vi "460 proj alpha.vi"() -> ()   [LabVIEW 2022 SP3]
uses:
  4060timecase.ctl
  <vilib>/sound2/lvsound2.llb/Sampling Mode.ctl
  4060subcasev2.ctl
  <vilib>/DAQmx/write.llb/DAQmx Write (Digital 1D Bool 1Chan 1Samp).vi
  62f802e7-f2dc-4d8a-a8e5-ab53cfb57c08.vi
  e1d0f7a0-9947-4ad8-8ac9-96135730a529.vi
  715f9e0f-8cb6-4fff-8a35-6535642fb82b.vi
  d1fa0bc4-31c7-44d2-9494-ddc12c5262e6.vi
  e97d7d1c-9cf7-499a-84b2-3041ff66f3d3.vi
  daa3e593-bf9d-4693-a451-b37ae69cdf9d.vi
  ae99be6c-c37c-4ad1-810a-db7e2be311bb.vi
  7a178aea-8366-4402-91cf-f9756686beea.vi
  5c64ab0a-a384-4fd4-873d-7fa8e23df335.vi
  1a855142-eefd-40c8-a2f9-4711cbabd8ad.vi
  aaa2aacd-ac84-4a8d-9874-ed439ef16769.vi
  2e93e64d-414c-47cd-bdfc-17e5d0d425ac.vi
  <vilib>/DAQmx/create/channels.llb/DAQmx Create Channel (DO-Digital Output).vi
  <vilib>/DAQmx/miscellaneous.llb/DAQmx Fill In Error Info.vi
  <vilib>/sound2/lvsound2.llb/Sound File Info (path).vi
  <vilib>/sound2/lvsound2.llb/Sound File Read Open.vi
  <vilib>/sound2/lvsound2.llb/Sound File Read (DBL).vi
  <vilib>/sound2/lvsound2.llb/Sound Output Write (DBL).vi
panel:
  out "error out 51":errorcluster
  out "error out 50":errorcluster
  out "error out 49":errorcluster
  out "error out 48":errorcluster
  out "error out 47":errorcluster
  out "error out 46":errorcluster
  out "error out 45":errorcluster
  out "error out 44":errorcluster
  out "error out 43":errorcluster
  out "error out 42":errorcluster
  out "error out 41":errorcluster
  out "error out 40":errorcluster
  out "error out 39":errorcluster
  in  "Number of Samples/Iteration":i32=2500
  in  "Device ID":u32
  in  "Stop":bool
  out "Current Iteration":i32
  out "Array 3":dbl[](array[numeric])
  out "Waveform Chart":waveform(dbl)[](graph)
  out "Array 7":bool[](array[boolean])
  out "error out 38":errorcluster
  out "error out 29":errorcluster
  out "Boolean 5":bool
  out "error out 25":errorcluster
  out "Boolean 4":bool
  out "Boolean 3":bool
  out "Boolean 2":bool
  out "error out 37":errorcluster
  out "error out 36":errorcluster
  out "error out 35":errorcluster
  out "error out 34":errorcluster
  out "error out 33":errorcluster
  out "error out 32":errorcluster
  out "error out 31":errorcluster
  out "error out 30":errorcluster
  out "error out 28":errorcluster
  out "error out 27":errorcluster
  out "error out 26":errorcluster
  in  "stop 3":bool
  # "I love those J I N G L E Bells\n\nOH\n\nThose Holiday J I N G L E Bells\n\nOH\n\nThose Happy J I N G L E\n\nB E double L S\n\nI love those J I N G L E bells\n\nOH\n\nJingle bells, jingle bells\n\nJingle all the way\n\nOh, what fun it is to ride\n\nIn a one horse open sleigh\n\nJingle bells, jingle bells\n\nJingle all the way\n\nOh, what fun it is to ride\n\nIn a one horse open sleigh\n\nDashing through the snow\n\n(Rudolph)\n\nIn a one horse open sleigh \n\n(Today)\n\nO'er the fields we go\n\n(Rudolph)\n\nLaughing all the way \n\n(Today)\n\nBells on bob-tail ring\n\nBING BING\n\nMakin' our spirits bright\n\nBONG BONG \n\nWhat fun it is to ride and sing\n\nA sleighin' song tonight\n\nHO HO HO\n\nHO HO HO\n\nHO HO HO HO HO\n\nHO HO HO HO HO HO HO\n \nHO HO HO HO HO HO\n\nJingle bells, jingle bells\n\nJingle all the way\n\nOh, what fun it is to ride\n\nIn a one horse open sleigh\n\nI love those J I N G L E Bells\n\nOH\n\nThose Holiday J I N G L E Bells\n\nOH\n\nThose Happy J I N G L E\n\nB E double L S\n\nI love those jingle bells\n\nAll the way!\n\nJingle all the\n\nWayyyyyyyyyy!"
  # "1. (v1)  0, 2, 4, (0 2 4 6), (1 3 5 7), (0 2 4 6), (1 3 5 7), (0 2 4 6), (1 3 5 7), off, \n\n(v1) LIGHTS\n\n(v2) 7, 5, 3, 1,  (1 3 5 7),  (0 2 4 6), (1 3 5 7),  (0 2 4 6),(1 3 5 7),  (0 2 4 6), off\n\n(v2) LIGHTS\n\n(v3)  0, 2, 4, (0 2 4 6), (1 3 5 7), (0 2 4 6), (1 3 5 7), (0 2 4 6), (1 3 5 7), off,\n\n2. (v4) (0 1), (7 6), off, (2 3), (4 5)\n\n(v5)  0, 2, 4, (0 2 4 6), (1 3 5 7), (0 2 4 6), (1 3 5 7), (0 2 4 6), (1 3 5 7), off\n\n(v6) LIGHTS"
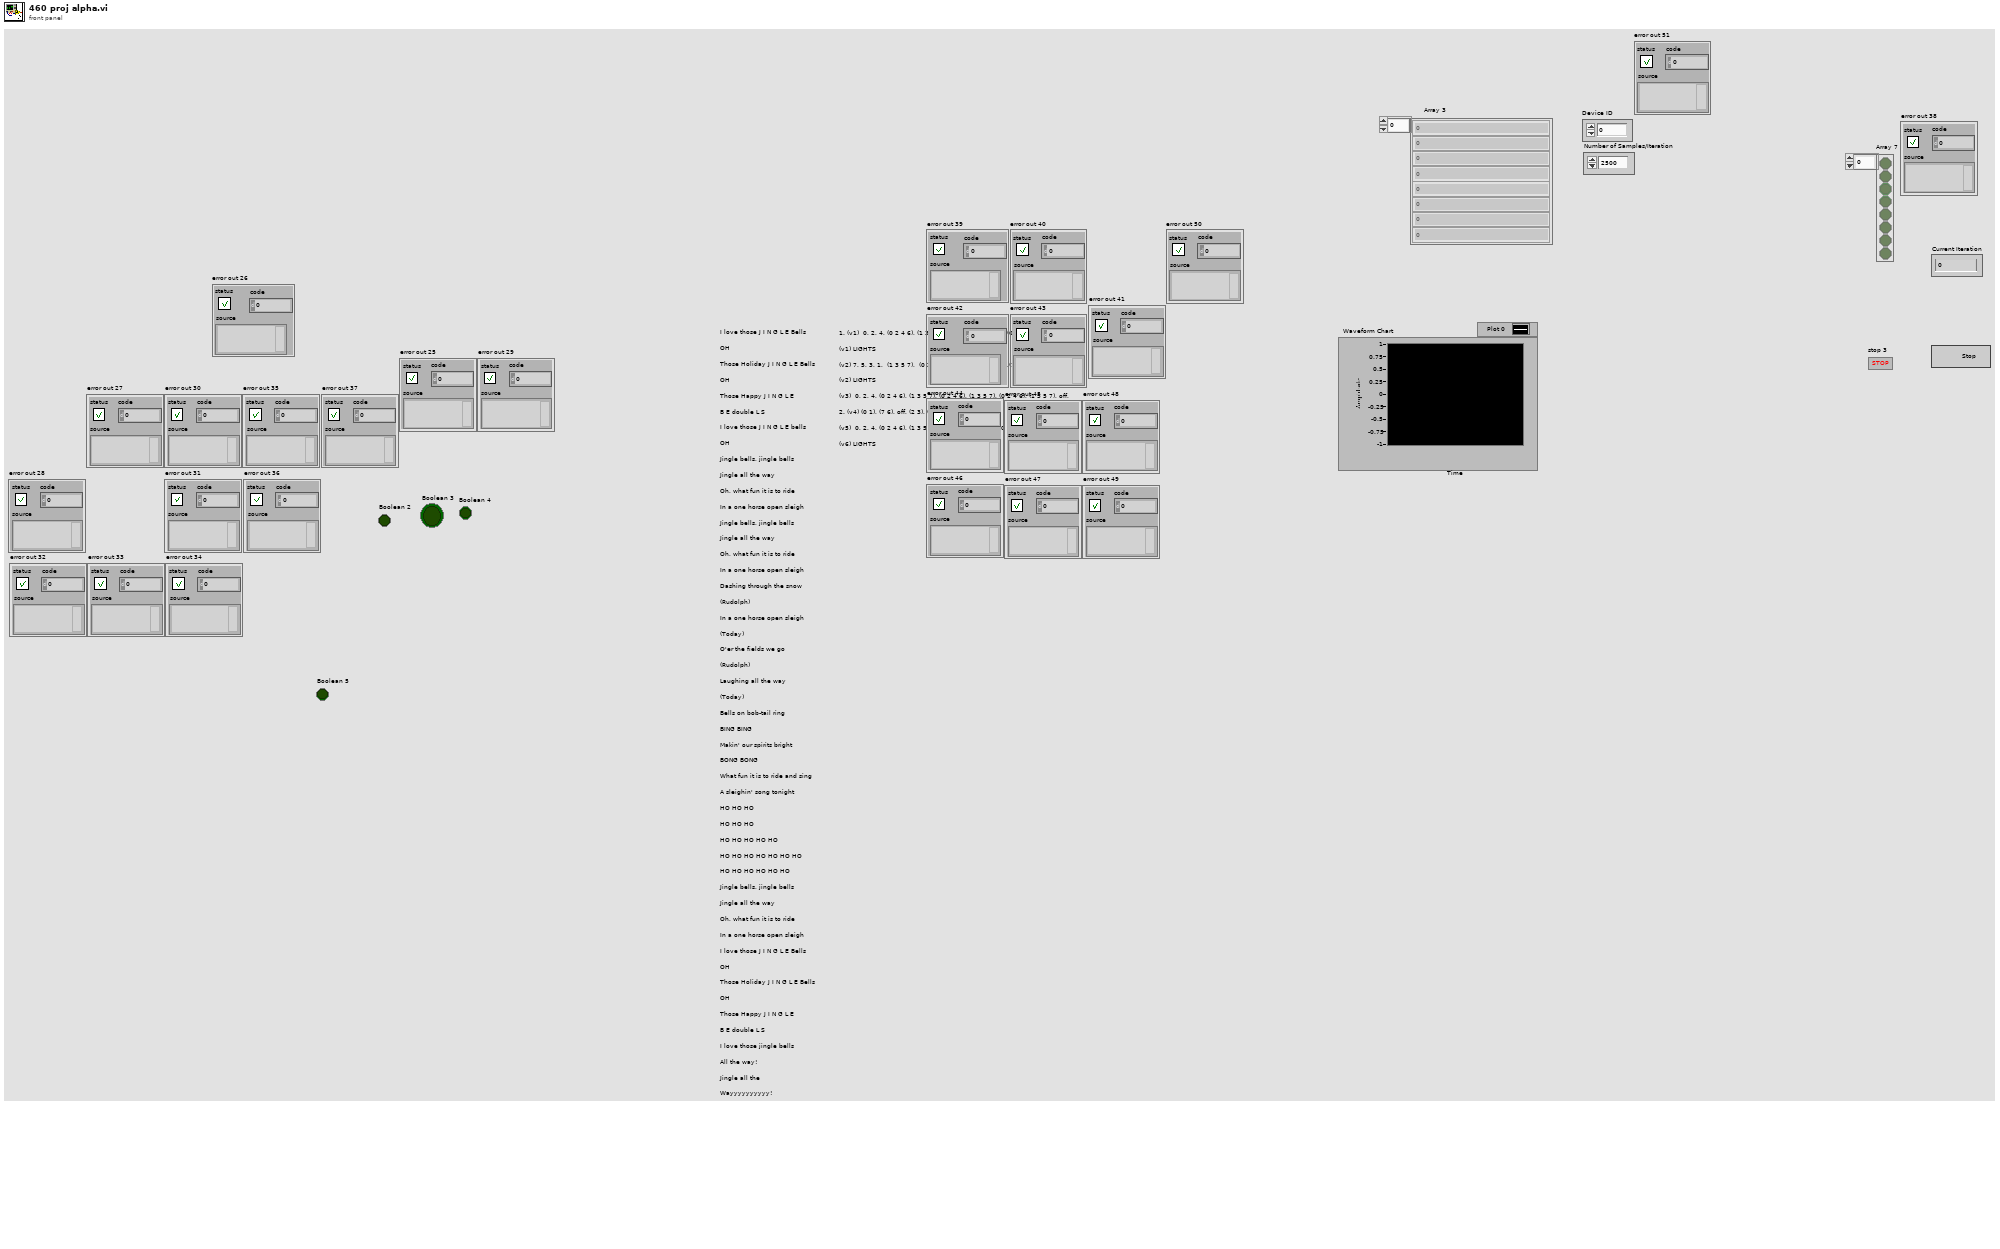
[diagram p1: front panel]
types:
  T1 = typedef "Sampling Mode.ctl" = i32
  T2 = typedef "4060timecase.ctl" = enum16{"v1-I love those", "v1-J", "v1-I", "v1-N", "v1-G", "v1-L", "v1-E", "v1-Bells", "v1-OH", "v1-OHoff", "v2-those holiday", "v2-J", "v2-I", "v2-N", "v2-G", "v2-L", "v2-E", "v2-Bells", "v2-OH", "v2-OHoff", "v3-those happy", "v3-J", "v3-I", "v3-N", "v3-G", "v3-L", "v3-E", "v4-B", "v4-E", "v4-double", "v4-L", "v4-S", "v4-Soff", "v5-I love those", "v5-J", "v5-I", "v5-N", "v5-G", "v5-L", "v5-E", "v5-Bells", "v5-OH", "v1-end"}
  T3 = typedef "4060subcasev2.ctl" = enum16{"v4 B", "v4 E", "v4 double", "v4 L", "v4 S", "v3 those happy", "off", "(0 2 4 6)", "LIGHTS", "(1 3 5 7)", "v1 I love those", "v2 those holiday"}
  T4 = typedef "Sound Data Format.ctl" = cluster{"sample rate (S/s)":dbl, "number of channels":i32, "bits per sample":i32}
  T5 = typedef "Sound File Refnum.ctl" = refnum<file>
  T6 = typedef "Sound Output Task ID.ctl" = u32
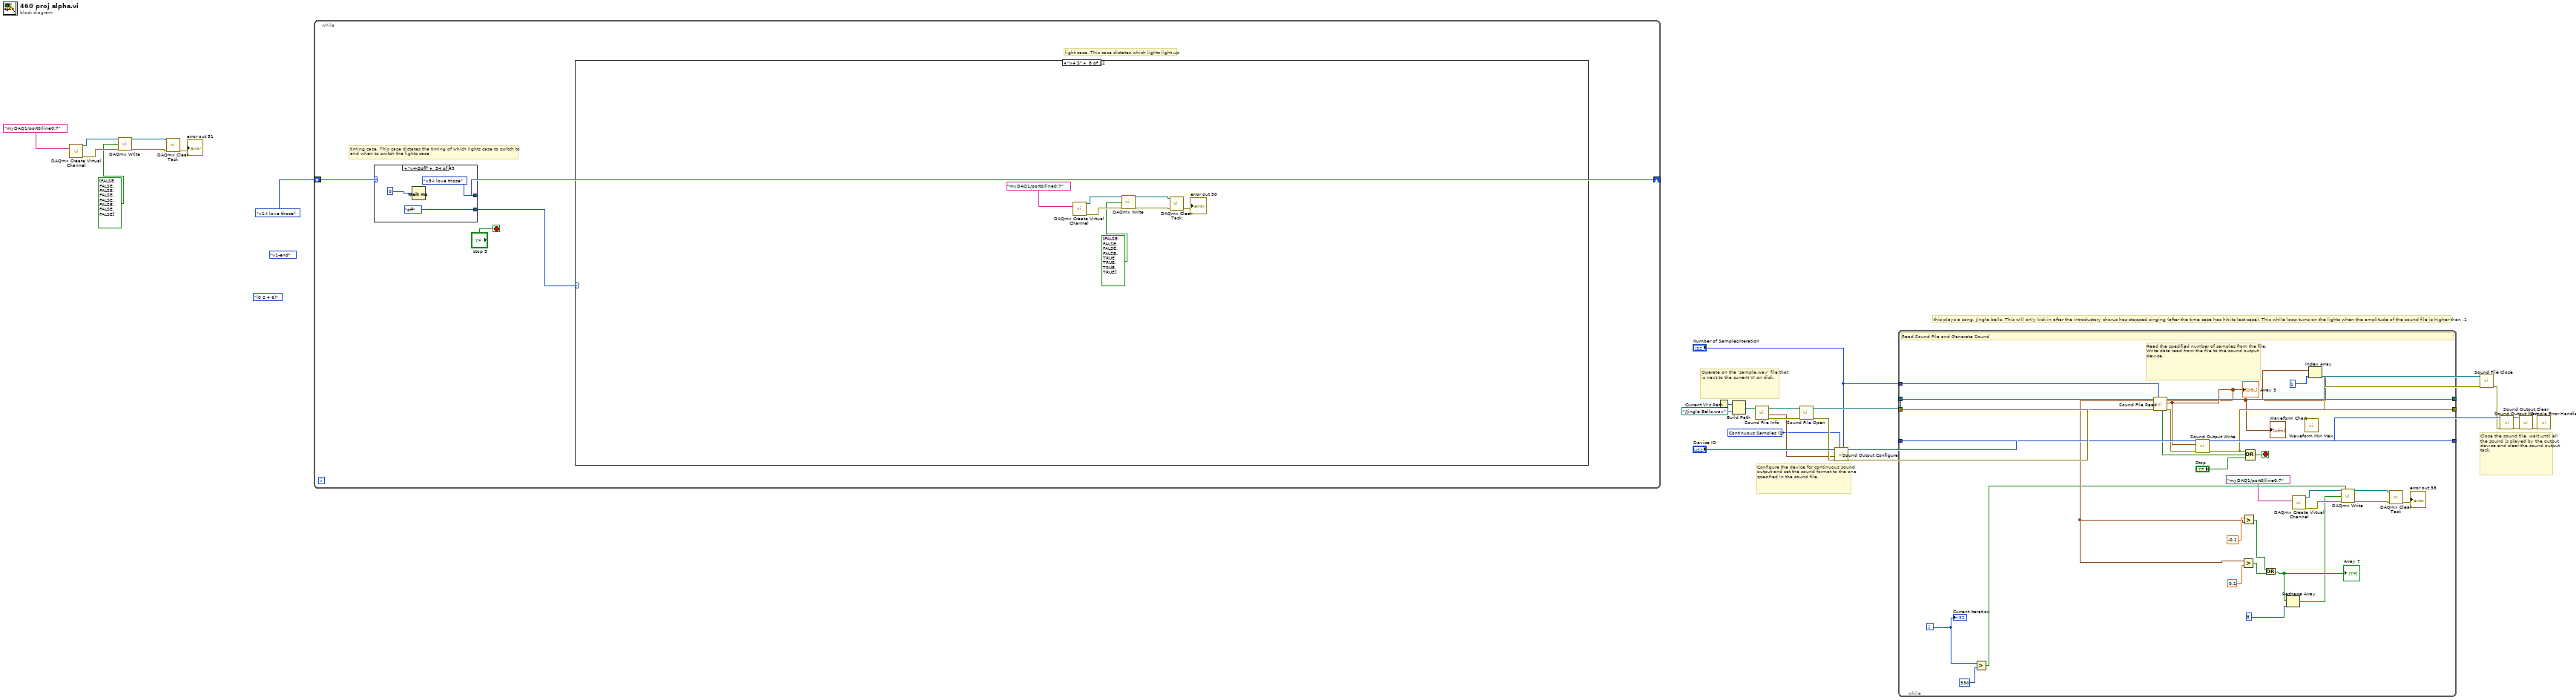
[diagram p0: block diagram]
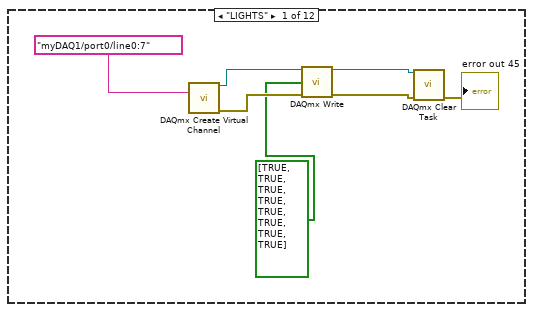
[diagram p2: hidden frame]
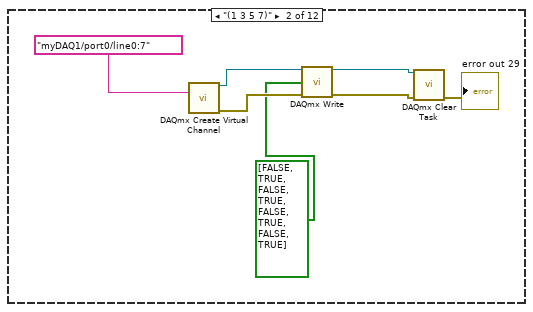
[diagram p3: hidden frame]
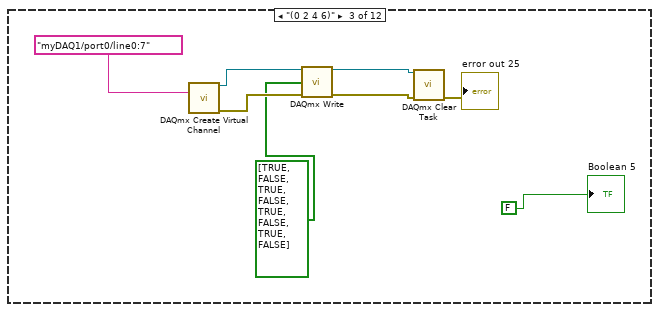
[diagram p4: hidden frame]
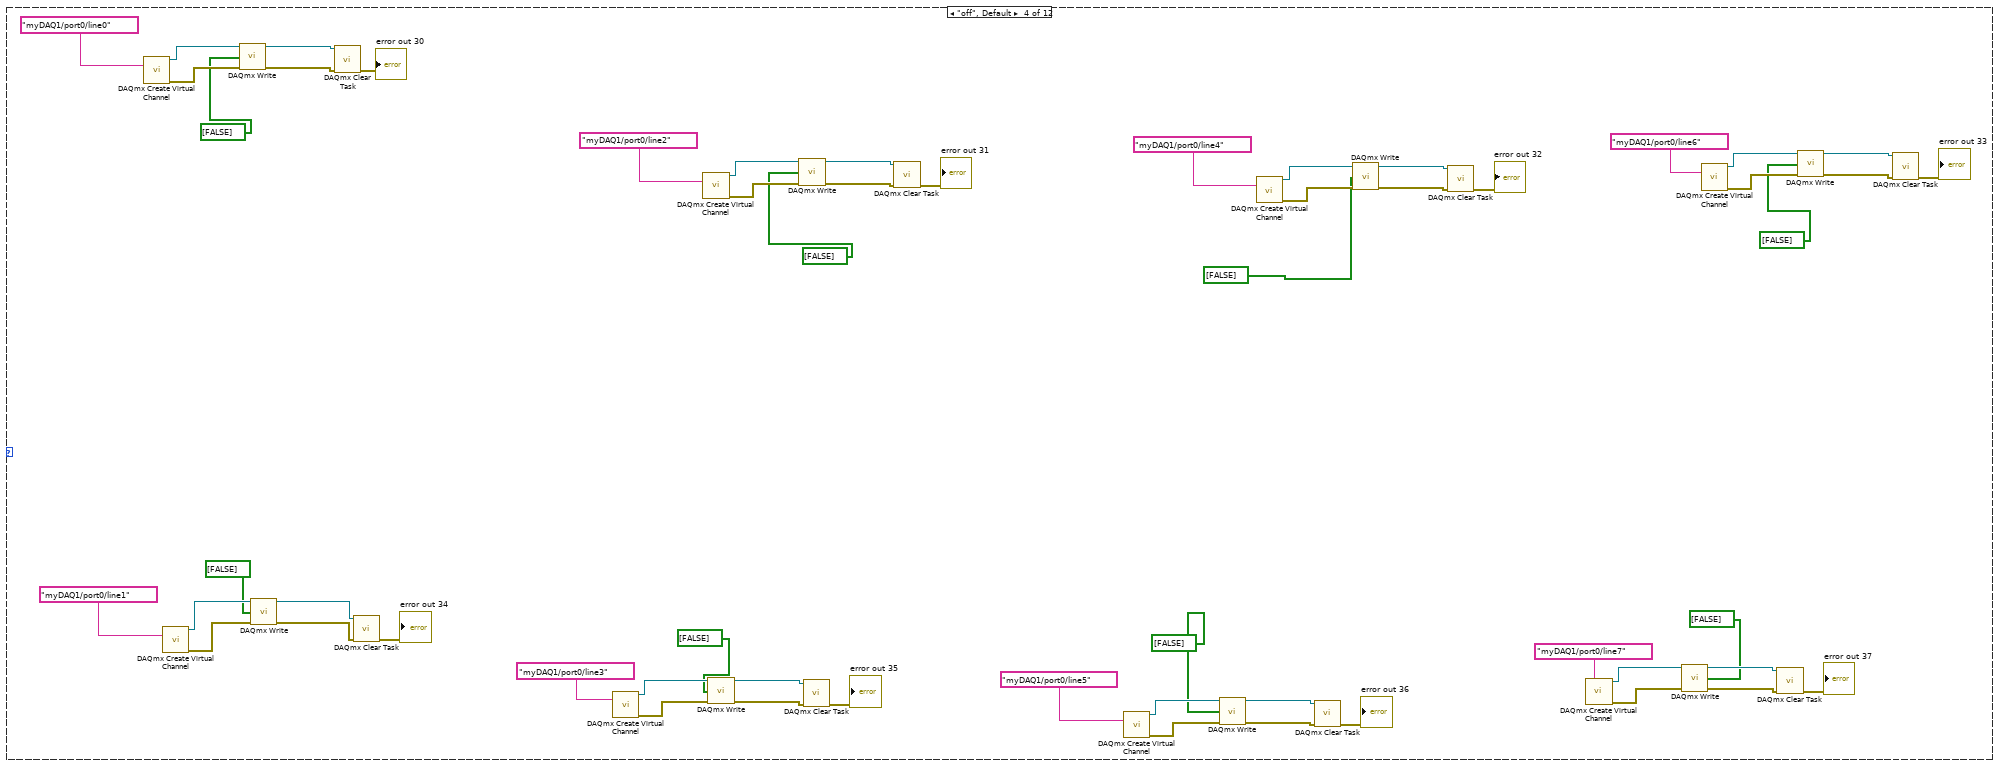
[diagram p5: hidden frame]
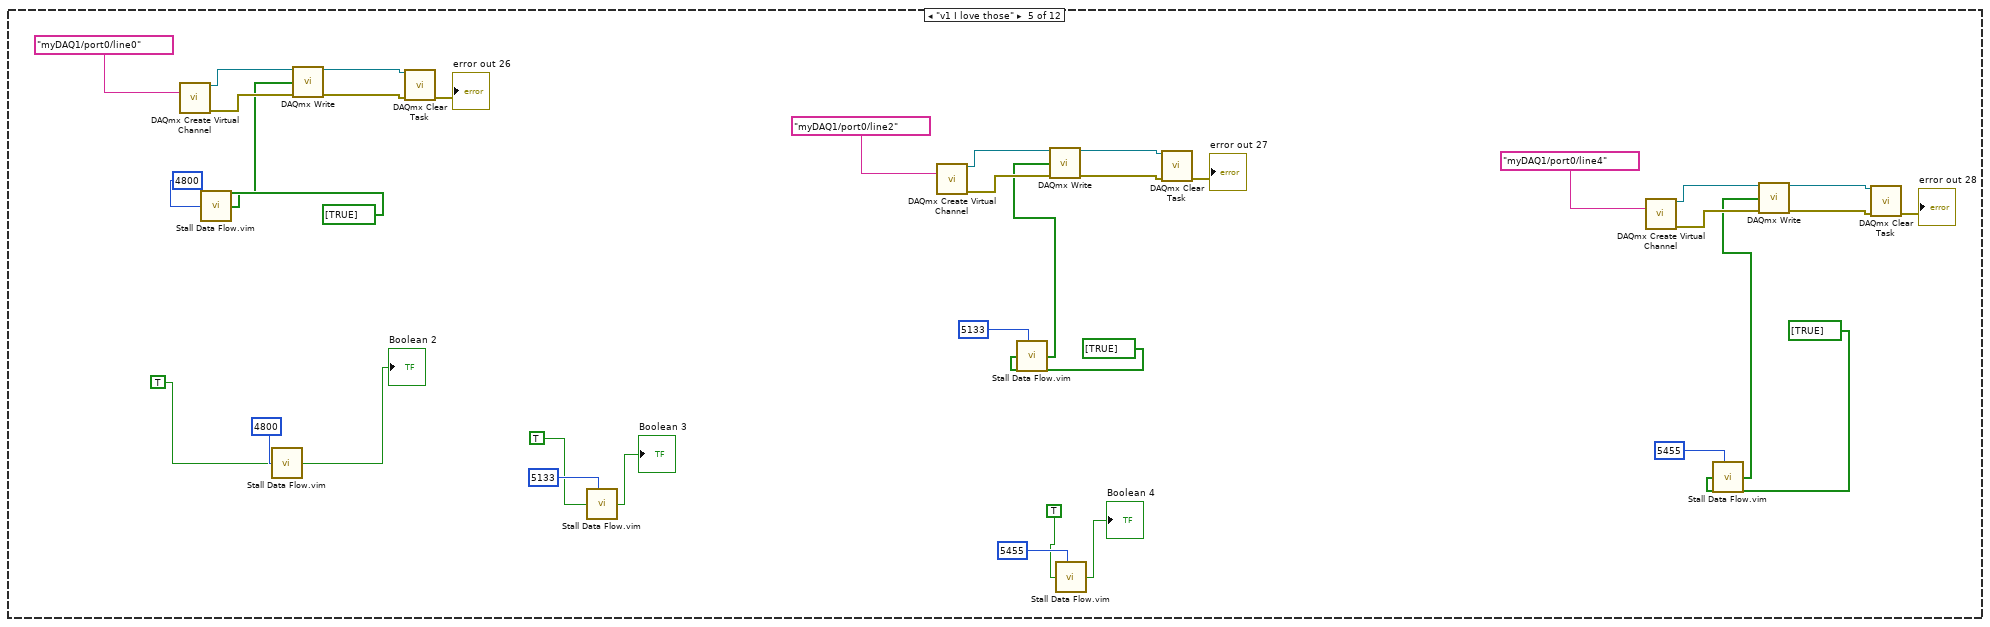
[diagram p6: hidden frame]
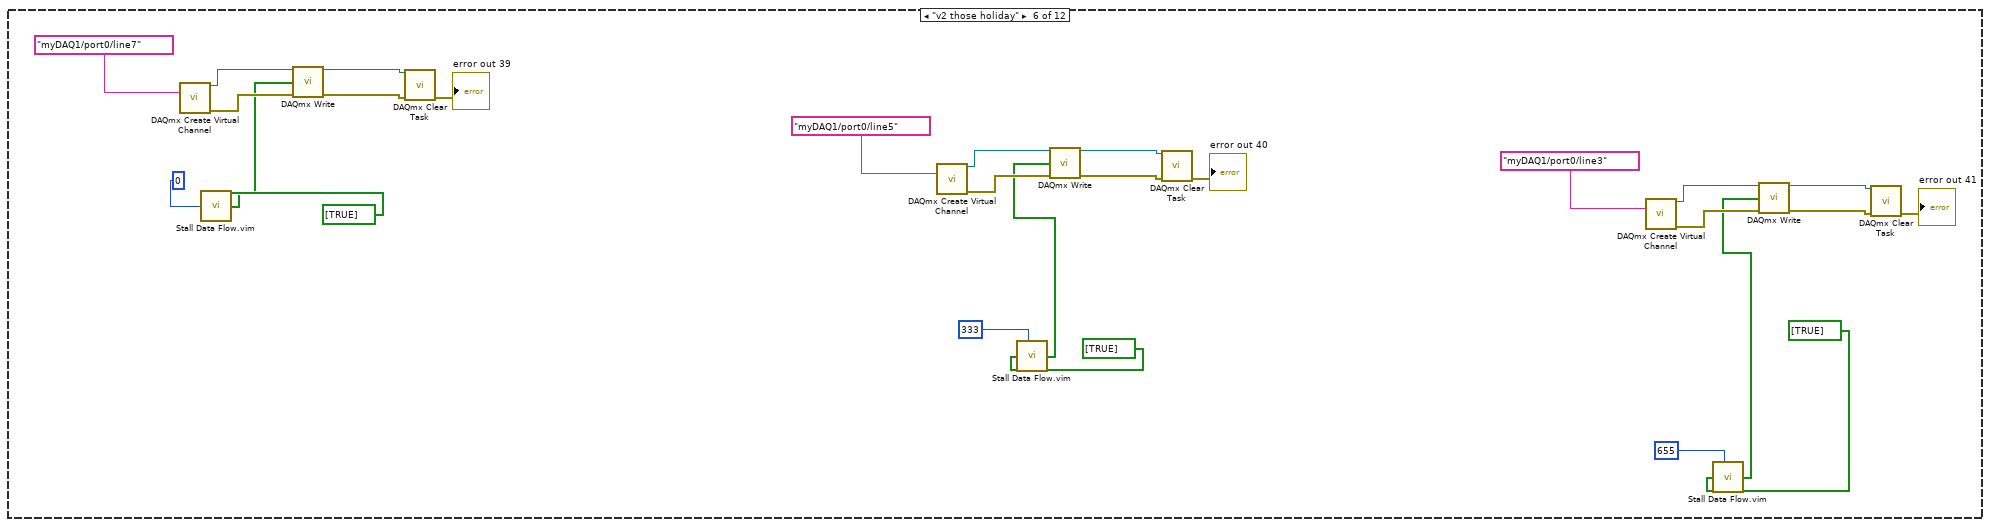
[diagram p7: hidden frame]
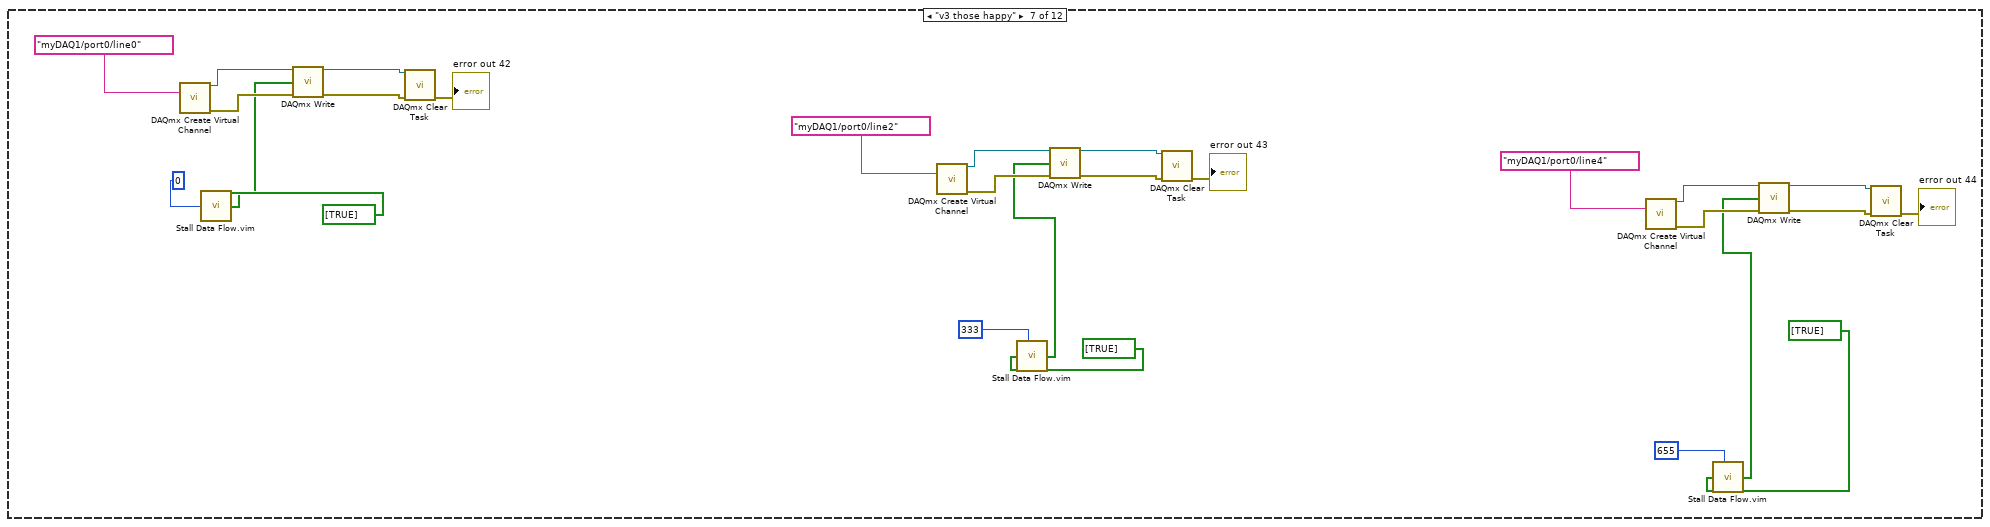
[diagram p8: hidden frame]
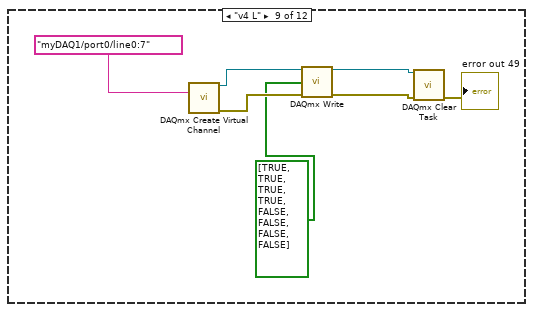
[diagram p9: hidden frame]
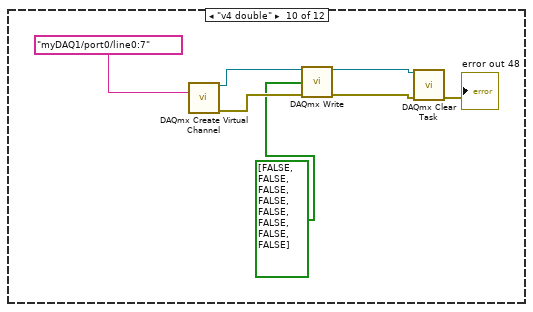
[diagram p10: hidden frame]
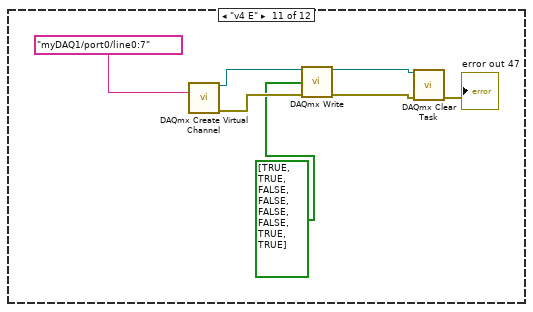
[diagram p11: hidden frame]
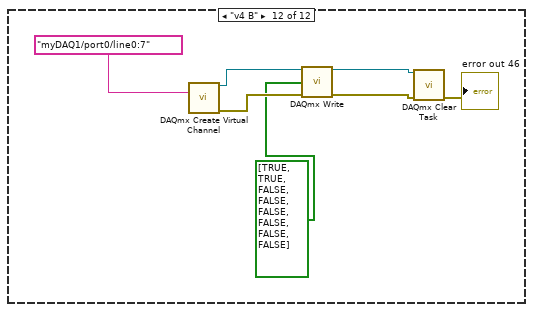
[diagram p12: hidden frame]
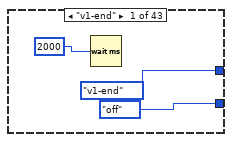
[diagram p13: hidden frame]
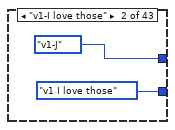
[diagram p14: hidden frame]
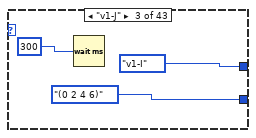
[diagram p15: hidden frame]
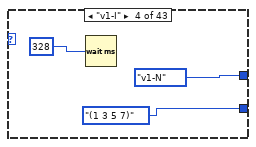
[diagram p16: hidden frame]
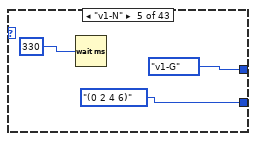
[diagram p17: hidden frame]
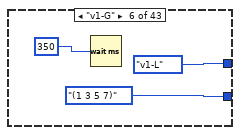
[diagram p18: hidden frame]
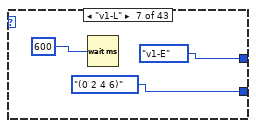
[diagram p19: hidden frame]
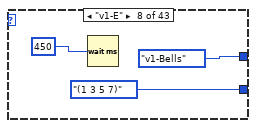
[diagram p20: hidden frame]
diagram:
  w12 = T1 1 items=["Finite Samples", "Continuous Samples"] ("sample mode")
  (unwired) 4060timecase."v1-end"
  (unwired) 4060subcasev2."(0 2 4 6)"
  # "this plays a song, Jingle bells. This will only kick in after the introductory chorus has stopped singing (after the time case has hit its last case). This while loop turns on the lights when the amplitude of the sound file is higher than .1"
  # "Operate on the 'sample.wav' file that is next to the current VI on disk."
  # "Close the sound file, wait until all the sound is played by the output device and clear the sound output task."
  # "Configure the device for continuous sound output and set the sound format to the one specified in the sound file."
  n1 = call-poly <vilib>:"DAQmx Create Virtual Channel.vi"("lines"=tag "myDAQ1/port0/line0:7") -> ("task out"=w7:refnum<k21>, "error out"=w5:errorcluster)  [unwired: 13 in]
  n2 = call-poly <vilib>:"DAQmx Write.vi"("task/channels in"=w7, "data"=bool[] [FALSE, FALSE, FALSE, FALSE, FALSE, FALSE, FALSE, FALSE], "error in"=w5) -> ("task out"=w6:refnum<k21>, "error out"=w4:errorcluster)  [unwired: 10 in, 1 out]
  n3 = call <vilib>:"DAQmx Clear Task.vi"("task in"=w6, "error in"=w4) -> ("error out"=→"error out 51":errorcluster)  [unwired: 13 in]
  n4 = while {
    shift-right: [w30] -> _
    shift-left: 4060timecase."v1-I love those" -> [w32]
    stop <- "stop 3" stop-if-true
    # "light case. This case dictates which lights light up"
    # "timing case. This case dictates the timing of which lights case to switch to\nand when to switch the lights case"
    n5 = case shown="\"v4-Soff\"" w32 {
      tunnel: [4060subcasev2."off" 4060subcasev2."v1 I love those" 4060subcasev2."(0 2 4 6)" 4060subcasev2."(1 3 5 7)" 4060subcasev2."(0 2 4 6)" 4060subcasev2."(1 3 5 7)" 4060subcasev2."(0 2 4 6)" 4060subcasev2."(1 3 5 7)" 4060subcasev2."off" 4060subcasev2."LIGHTS" 4060subcasev2."off" 4060subcasev2."v2 those holiday" 4060subcasev2."(1 3 5 7)" 4060subcasev2."(0 2 4 6)" 4060subcasev2."(1 3 5 7)" 4060subcasev2."(0 2 4 6)" 4060subcasev2."(1 3 5 7)" 4060subcasev2."(0 2 4 6)" 4060subcasev2."off" 4060subcasev2."LIGHTS" 4060subcasev2."off" 4060subcasev2."v3 those happy" 4060subcasev2."(0 2 4 6)" 4060subcasev2."(1 3 5 7)" 4060subcasev2."(0 2 4 6)" 4060subcasev2."(1 3 5 7)" 4060subcasev2."(0 2 4 6)" 4060subcasev2."(1 3 5 7)" 4060subcasev2."v4 B" 4060subcasev2."v4 E" 4060subcasev2."v4 double" 4060subcasev2."v4 L" 4060subcasev2."v4 S" 4060subcasev2."off" 4060subcasev2."v2 those holiday" 4060subcasev2."(1 3 5 7)" 4060subcasev2."(0 2 4 6)" 4060subcasev2."(1 3 5 7)" 4060subcasev2."(0 2 4 6)" 4060subcasev2."(1 3 5 7)" 4060subcasev2."(0 2 4 6)" 4060subcasev2."off" 4060subcasev2."LIGHTS"] -> w29
      tunnel: [4060timecase."v1-end" 4060timecase."v1-J" 4060timecase."v1-I" 4060timecase."v1-N" 4060timecase."v1-G" 4060timecase."v1-L" 4060timecase."v1-E" 4060timecase."v1-Bells" 4060timecase."v1-OH" 4060timecase."v1-OHoff" 4060timecase."v2-those holiday" 4060timecase."v2-J" 4060timecase."v2-I" 4060timecase."v2-N" 4060timecase."v2-G" 4060timecase."v2-L" 4060timecase."v2-E" 4060timecase."v2-Bells" 4060timecase."v2-OH" 4060timecase."v2-OHoff" 4060timecase."v3-those happy" 4060timecase."v3-J" 4060timecase."v3-I" 4060timecase."v3-N" 4060timecase."v3-G" 4060timecase."v3-L" 4060timecase."v3-E" 4060timecase."v4-B" 4060timecase."v4-E" 4060timecase."v4-double" 4060timecase."v4-L" 4060timecase."v4-S" 4060timecase."v4-Soff" 4060timecase."v5-I love those" 4060timecase."v5-J" 4060timecase."v5-I" 4060timecase."v5-N" 4060timecase."v5-G" 4060timecase."v5-L" 4060timecase."v5-E" 4060timecase."v5-Bells" 4060timecase."v5-OH" 4060timecase."v1-end"] -> w30
      frame "v1-end" {
        n6 = Wait (ms)(milliseconds to wait=2000) -> ()  [unwired: 1 out]
      }
      frame "v1-I love those" {
      }
      frame "v1-J" {
        n7 = Wait (ms)(milliseconds to wait=300) -> ()  [unwired: 1 out]
      }
      frame "v1-I" {
        n8 = Wait (ms)(milliseconds to wait=328) -> ()  [unwired: 1 out]
      }
      frame "v1-N" {
        n9 = Wait (ms)(milliseconds to wait=330) -> ()  [unwired: 1 out]
      }
      frame "v1-G" {
        n10 = Wait (ms)(milliseconds to wait=350) -> ()  [unwired: 1 out]
      }
      frame "v1-L" {
        n11 = Wait (ms)(milliseconds to wait=600) -> ()  [unwired: 1 out]
      }
      frame "v1-E" {
        n12 = Wait (ms)(milliseconds to wait=450) -> ()  [unwired: 1 out]
      }
      frame "v1-Bells" {
        n13 = Wait (ms)(milliseconds to wait=330) -> ()  [unwired: 1 out]
      }
      frame "v1-OH" {
        n14 = Wait (ms)(milliseconds to wait=1000) -> ()  [unwired: 1 out]
      }
      frame "v1-OHoff" {
        n15 = Wait (ms)(milliseconds to wait=300) -> ()  [unwired: 1 out]
      }
      frame "v2-those holiday" {
        n16 = Wait (ms)(milliseconds to wait=500) -> ()  [unwired: 1 out]
      }
      frame "v2-J" {
        n17 = Wait (ms)(milliseconds to wait=300) -> ()  [unwired: 1 out]
      }
      frame "v2-I" {
        n18 = Wait (ms)(milliseconds to wait=328) -> ()  [unwired: 1 out]
      }
      frame "v2-N" {
        n19 = Wait (ms)(milliseconds to wait=330) -> ()  [unwired: 1 out]
      }
      frame "v2-G" {
        n20 = Wait (ms)(milliseconds to wait=350) -> ()  [unwired: 1 out]
      }
      frame "v2-L" {
        n21 = Wait (ms)(milliseconds to wait=600) -> ()  [unwired: 1 out]
      }
      frame "v2-E" {
        n22 = Wait (ms)(milliseconds to wait=450) -> ()  [unwired: 1 out]
      }
      frame "v2-Bells" {
        n23 = Wait (ms)(milliseconds to wait=330) -> ()  [unwired: 1 out]
      }
      frame "v2-OH" {
        n24 = Wait (ms)(milliseconds to wait=1000) -> ()  [unwired: 1 out]
      }
      frame "v2-OHoff" {
        n25 = Wait (ms)(milliseconds to wait=300) -> ()  [unwired: 1 out]
      }
      frame "v3-those happy" {
        n26 = Wait (ms)(milliseconds to wait=330) -> ()  [unwired: 1 out]
      }
      frame "v3-J" {
        n27 = Wait (ms)(milliseconds to wait=330) -> ()  [unwired: 1 out]
      }
      frame "v3-I" {
        n28 = Wait (ms)(milliseconds to wait=328) -> ()  [unwired: 1 out]
      }
      frame "v3-N" {
        n29 = Wait (ms)(milliseconds to wait=330) -> ()  [unwired: 1 out]
      }
      frame "v3-G" {
        n30 = Wait (ms)(milliseconds to wait=350) -> ()  [unwired: 1 out]
      }
      frame "v3-L" {
        n31 = Wait (ms)(milliseconds to wait=600) -> ()  [unwired: 1 out]
      }
      frame "v3-E" {
        n32 = Wait (ms)(milliseconds to wait=450) -> ()  [unwired: 1 out]
      }
      frame "v4-B" {
        n33 = Wait (ms)(milliseconds to wait=1000) -> ()  [unwired: 1 out]
      }
      frame "v4-E" {
        n34 = Wait (ms)(milliseconds to wait=330) -> ()  [unwired: 1 out]
      }
      frame "v4-double" {
        n35 = Wait (ms)(milliseconds to wait=330) -> ()  [unwired: 1 out]
      }
      frame "v4-L" {
        n36 = Wait (ms)(milliseconds to wait=330) -> ()  [unwired: 1 out]
      }
      frame "v4-S" {
        n37 = Wait (ms)(milliseconds to wait=330) -> ()  [unwired: 1 out]
      }
      frame "v4-Soff" {
        n38 = Wait (ms)(milliseconds to wait=0) -> ()  [unwired: 1 out]
      }
      frame "v5-I love those" {
        n39 = Wait (ms)(milliseconds to wait=330) -> ()  [unwired: 1 out]
      }
      frame "v5-J" {
        n40 = Wait (ms)(milliseconds to wait=330) -> ()  [unwired: 1 out]
      }
      frame "v5-I" {
        n41 = Wait (ms)(milliseconds to wait=330) -> ()  [unwired: 1 out]
      }
      frame "v5-N" {
        n42 = Wait (ms)(milliseconds to wait=330) -> ()  [unwired: 1 out]
      }
      frame "v5-G" {
        n43 = Wait (ms)(milliseconds to wait=330) -> ()  [unwired: 1 out]
      }
      frame "v5-L" {
        n44 = Wait (ms)(milliseconds to wait=330) -> ()  [unwired: 1 out]
      }
      frame "v5-E" {
        n45 = Wait (ms)(milliseconds to wait=330) -> ()  [unwired: 1 out]
      }
      frame "v5-Bells" {
        n46 = Wait (ms)(milliseconds to wait=330) -> ()  [unwired: 1 out]
      }
      frame "v5-OH" {
        n47 = Wait (ms)(milliseconds to wait=330) -> ()  [unwired: 1 out]
      }
    }
    n48 = case shown="\"v4 S\"" w29 {
      frame "LIGHTS" {
        n49 = call-poly <vilib>:"DAQmx Create Virtual Channel.vi"("lines"=tag "myDAQ1/port0/line0:7") -> ("task out"=w39:refnum<k21>, "error out"=w37:errorcluster)  [unwired: 13 in]
        n50 = call-poly <vilib>:"DAQmx Write.vi"("task/channels in"=w39, "data"=bool[] [TRUE, TRUE, TRUE, TRUE, TRUE, TRUE, TRUE, TRUE], "error in"=w37) -> ("task out"=w38:refnum<k21>, "error out"=w36:errorcluster)  [unwired: 10 in, 1 out]
        n51 = call <vilib>:"DAQmx Clear Task.vi"("task in"=w38, "error in"=w36) -> ("error out"=→"error out 45":errorcluster)  [unwired: 13 in]
      }
      frame "(1 3 5 7)" {
        n52 = call-poly <vilib>:"DAQmx Create Virtual Channel.vi"("lines"=tag "myDAQ1/port0/line0:7") -> ("task out"=w46:refnum<k21>, "error out"=w44:errorcluster)  [unwired: 13 in]
        n53 = call-poly <vilib>:"DAQmx Write.vi"("task/channels in"=w46, "data"=bool[] [FALSE, TRUE, FALSE, TRUE, FALSE, TRUE, FALSE, TRUE], "error in"=w44) -> ("task out"=w45:refnum<k21>, "error out"=w43:errorcluster)  [unwired: 10 in, 1 out]
        n54 = call <vilib>:"DAQmx Clear Task.vi"("task in"=w45, "error in"=w43) -> ("error out"=→"error out 29":errorcluster)  [unwired: 13 in]
      }
      frame "(0 2 4 6)" {
        n55 = call-poly <vilib>:"DAQmx Create Virtual Channel.vi"("lines"=tag "myDAQ1/port0/line0:7") -> ("task out"=w54:refnum<k21>, "error out"=w52:errorcluster)  [unwired: 13 in]
        n56 = call-poly <vilib>:"DAQmx Write.vi"("task/channels in"=w54, "data"=bool[] [TRUE, FALSE, TRUE, FALSE, TRUE, FALSE, TRUE, FALSE], "error in"=w52) -> ("task out"=w53:refnum<k21>, "error out"=w51:errorcluster)  [unwired: 10 in, 1 out]
        n57 = call <vilib>:"DAQmx Clear Task.vi"("task in"=w53, "error in"=w51) -> ("error out"=→"error out 25":errorcluster)  [unwired: 13 in]
        "Boolean 5" <- FALSE
      }
      frame "off", Default {
        n58 = call-poly <vilib>:"DAQmx Create Virtual Channel.vi"("lines"=tag "myDAQ1/port0/line0") -> ("task out"=w110:refnum<k21>, "error out"=w108:errorcluster)  [unwired: 13 in]
        n59 = call-poly <vilib>:"DAQmx Create Virtual Channel.vi"("lines"=tag "myDAQ1/port0/line1") -> ("task out"=w86:refnum<k21>, "error out"=w84:errorcluster)  [unwired: 13 in]
        n60 = call-poly <vilib>:"DAQmx Write.vi"("task/channels in"=w110, "data"=bool[] [FALSE], "error in"=w108) -> ("task out"=w109:refnum<k21>, "error out"=w107:errorcluster)  [unwired: 10 in, 1 out]
        n61 = call-poly <vilib>:"DAQmx Write.vi"("task/channels in"=w86, "data"=bool[] [FALSE], "error in"=w84) -> ("task out"=w85:refnum<k21>, "error out"=w83:errorcluster)  [unwired: 10 in, 1 out]
        n62 = call <vilib>:"DAQmx Clear Task.vi"("task in"=w109, "error in"=w107) -> ("error out"=→"error out 30":errorcluster)  [unwired: 13 in]
        n63 = call <vilib>:"DAQmx Clear Task.vi"("task in"=w85, "error in"=w83) -> ("error out"=→"error out 34":errorcluster)  [unwired: 13 in]
        n64 = call-poly <vilib>:"DAQmx Create Virtual Channel.vi"("lines"=tag "myDAQ1/port0/line3") -> ("task out"=w80:refnum<k21>, "error out"=w78:errorcluster)  [unwired: 13 in]
        n65 = call-poly <vilib>:"DAQmx Create Virtual Channel.vi"("lines"=tag "myDAQ1/port0/line2") -> ("task out"=w104:refnum<k21>, "error out"=w102:errorcluster)  [unwired: 13 in]
        n66 = call-poly <vilib>:"DAQmx Write.vi"("task/channels in"=w80, "data"=bool[] [FALSE], "error in"=w78) -> ("task out"=w79:refnum<k21>, "error out"=w77:errorcluster)  [unwired: 10 in, 1 out]
        n67 = call-poly <vilib>:"DAQmx Write.vi"("task/channels in"=w104, "data"=bool[] [FALSE], "error in"=w102) -> ("task out"=w103:refnum<k21>, "error out"=w101:errorcluster)  [unwired: 10 in, 1 out]
        n68 = call <vilib>:"DAQmx Clear Task.vi"("task in"=w79, "error in"=w77) -> ("error out"=→"error out 35":errorcluster)  [unwired: 13 in]
        n69 = call <vilib>:"DAQmx Clear Task.vi"("task in"=w103, "error in"=w101) -> ("error out"=→"error out 31":errorcluster)  [unwired: 13 in]
        n70 = call-poly <vilib>:"DAQmx Create Virtual Channel.vi"("lines"=tag "myDAQ1/port0/line5") -> ("task out"=w74:refnum<k21>, "error out"=w72:errorcluster)  [unwired: 13 in]
        n71 = call-poly <vilib>:"DAQmx Write.vi"("task/channels in"=w74, "data"=bool[] [FALSE], "error in"=w72) -> ("task out"=w73:refnum<k21>, "error out"=w71:errorcluster)  [unwired: 10 in, 1 out]
        n72 = call-poly <vilib>:"DAQmx Create Virtual Channel.vi"("lines"=tag "myDAQ1/port0/line4") -> ("task out"=w98:refnum<k21>, "error out"=w96:errorcluster)  [unwired: 13 in]
        n73 = call <vilib>:"DAQmx Clear Task.vi"("task in"=w73, "error in"=w71) -> ("error out"=→"error out 36":errorcluster)  [unwired: 13 in]
        n74 = call-poly <vilib>:"DAQmx Write.vi"("task/channels in"=w98, "data"=bool[] [FALSE], "error in"=w96) -> ("task out"=w97:refnum<k21>, "error out"=w95:errorcluster)  [unwired: 10 in, 1 out]
        n75 = call <vilib>:"DAQmx Clear Task.vi"("task in"=w97, "error in"=w95) -> ("error out"=→"error out 32":errorcluster)  [unwired: 13 in]
        n76 = call-poly <vilib>:"DAQmx Create Virtual Channel.vi"("lines"=tag "myDAQ1/port0/line7") -> ("task out"=w68:refnum<k21>, "error out"=w66:errorcluster)  [unwired: 13 in]
        n77 = call-poly <vilib>:"DAQmx Write.vi"("task/channels in"=w68, "data"=bool[] [FALSE], "error in"=w66) -> ("task out"=w67:refnum<k21>, "error out"=w65:errorcluster)  [unwired: 10 in, 1 out]
        n78 = call-poly <vilib>:"DAQmx Create Virtual Channel.vi"("lines"=tag "myDAQ1/port0/line6") -> ("task out"=w92:refnum<k21>, "error out"=w90:errorcluster)  [unwired: 13 in]
        n79 = call <vilib>:"DAQmx Clear Task.vi"("task in"=w67, "error in"=w65) -> ("error out"=→"error out 37":errorcluster)  [unwired: 13 in]
        n80 = call-poly <vilib>:"DAQmx Write.vi"("task/channels in"=w92, "data"=bool[] [FALSE], "error in"=w90) -> ("task out"=w91:refnum<k21>, "error out"=w89:errorcluster)  [unwired: 10 in, 1 out]
        n81 = call <vilib>:"DAQmx Clear Task.vi"("task in"=w91, "error in"=w89) -> ("error out"=→"error out 33":errorcluster)  [unwired: 13 in]
      }
      frame "v1 I love those" {
        n82 = call-poly <vilib>:"DAQmx Create Virtual Channel.vi"("lines"=tag "myDAQ1/port0/line0") -> ("task out"=w146:refnum<k21>, "error out"=w144:errorcluster)  [unwired: 13 in]
        n83 = call "Stall Data Flow.vim"("value in"=bool[] [TRUE], "milliseconds to wait"=4800) -> ("value out"=w117:bool[])  [unwired: 1 out]
        n84 = call "Stall Data Flow.vim"("value in"=TRUE, "milliseconds to wait"=4800) -> ("value out"=→"Boolean 2":bool)  [unwired: 1 out]
        n85 = call-poly <vilib>:"DAQmx Write.vi"("task/channels in"=w146, "data"=w117, "error in"=w144) -> ("task out"=w145:refnum<k21>, "error out"=w143:errorcluster)  [unwired: 10 in, 1 out]
        n86 = call <vilib>:"DAQmx Clear Task.vi"("task in"=w145, "error in"=w143) -> ("error out"=→"error out 26":errorcluster)  [unwired: 13 in]
        n87 = call "Stall Data Flow.vim"("value in"=TRUE, "milliseconds to wait"=5133) -> ("value out"=→"Boolean 3":bool)  [unwired: 1 out]
        n88 = call-poly <vilib>:"DAQmx Create Virtual Channel.vi"("lines"=tag "myDAQ1/port0/line2") -> ("task out"=w140:refnum<k21>, "error out"=w138:errorcluster)  [unwired: 13 in]
        n89 = call "Stall Data Flow.vim"("value in"=bool[] [TRUE], "milliseconds to wait"=5133) -> ("value out"=w115:bool[])  [unwired: 1 out]
        n90 = call-poly <vilib>:"DAQmx Write.vi"("task/channels in"=w140, "data"=w115, "error in"=w138) -> ("task out"=w139:refnum<k21>, "error out"=w137:errorcluster)  [unwired: 10 in, 1 out]
        n91 = call "Stall Data Flow.vim"("value in"=TRUE, "milliseconds to wait"=5455) -> ("value out"=→"Boolean 4":bool)  [unwired: 1 out]
        n92 = call <vilib>:"DAQmx Clear Task.vi"("task in"=w139, "error in"=w137) -> ("error out"=→"error out 27":errorcluster)  [unwired: 13 in]
        n93 = call-poly <vilib>:"DAQmx Create Virtual Channel.vi"("lines"=tag "myDAQ1/port0/line4") -> ("task out"=w134:refnum<k21>, "error out"=w132:errorcluster)  [unwired: 13 in]
        n94 = call "Stall Data Flow.vim"("value in"=bool[] [TRUE], "milliseconds to wait"=5455) -> ("value out"=w112:bool[])  [unwired: 1 out]
        n95 = call-poly <vilib>:"DAQmx Write.vi"("task/channels in"=w134, "data"=w112, "error in"=w132) -> ("task out"=w133:refnum<k21>, "error out"=w131:errorcluster)  [unwired: 10 in, 1 out]
        n96 = call <vilib>:"DAQmx Clear Task.vi"("task in"=w133, "error in"=w131) -> ("error out"=→"error out 28":errorcluster)  [unwired: 13 in]
      }
      frame "v2 those holiday" {
        n97 = call-poly <vilib>:"DAQmx Create Virtual Channel.vi"("lines"=tag "myDAQ1/port0/line7") -> ("task out"=w173:refnum<k21>, "error out"=w171:errorcluster)  [unwired: 13 in]
        n98 = call "Stall Data Flow.vim"("value in"=bool[] [TRUE], "milliseconds to wait"=0) -> ("value out"=w153:bool[])  [unwired: 1 out]
        n99 = call-poly <vilib>:"DAQmx Write.vi"("task/channels in"=w173, "data"=w153, "error in"=w171) -> ("task out"=w172:refnum<k21>, "error out"=w170:errorcluster)  [unwired: 10 in, 1 out]
        n100 = call <vilib>:"DAQmx Clear Task.vi"("task in"=w172, "error in"=w170) -> ("error out"=→"error out 39":errorcluster)  [unwired: 13 in]
        n101 = call-poly <vilib>:"DAQmx Create Virtual Channel.vi"("lines"=tag "myDAQ1/port0/line5") -> ("task out"=w167:refnum<k21>, "error out"=w165:errorcluster)  [unwired: 13 in]
        n102 = call "Stall Data Flow.vim"("value in"=bool[] [TRUE], "milliseconds to wait"=333) -> ("value out"=w151:bool[])  [unwired: 1 out]
        n103 = call-poly <vilib>:"DAQmx Write.vi"("task/channels in"=w167, "data"=w151, "error in"=w165) -> ("task out"=w166:refnum<k21>, "error out"=w164:errorcluster)  [unwired: 10 in, 1 out]
        n104 = call <vilib>:"DAQmx Clear Task.vi"("task in"=w166, "error in"=w164) -> ("error out"=→"error out 40":errorcluster)  [unwired: 13 in]
        n105 = call-poly <vilib>:"DAQmx Create Virtual Channel.vi"("lines"=tag "myDAQ1/port0/line3") -> ("task out"=w161:refnum<k21>, "error out"=w159:errorcluster)  [unwired: 13 in]
        n106 = call "Stall Data Flow.vim"("value in"=bool[] [TRUE], "milliseconds to wait"=655) -> ("value out"=w148:bool[])  [unwired: 1 out]
        n107 = call-poly <vilib>:"DAQmx Write.vi"("task/channels in"=w161, "data"=w148, "error in"=w159) -> ("task out"=w160:refnum<k21>, "error out"=w158:errorcluster)  [unwired: 10 in, 1 out]
        n108 = call <vilib>:"DAQmx Clear Task.vi"("task in"=w160, "error in"=w158) -> ("error out"=→"error out 41":errorcluster)  [unwired: 13 in]
      }
      frame "v3 those happy" {
        n109 = call-poly <vilib>:"DAQmx Create Virtual Channel.vi"("lines"=tag "myDAQ1/port0/line0") -> ("task out"=w200:refnum<k21>, "error out"=w198:errorcluster)  [unwired: 13 in]
        n110 = call "Stall Data Flow.vim"("value in"=bool[] [TRUE], "milliseconds to wait"=0) -> ("value out"=w180:bool[])  [unwired: 1 out]
        n111 = call-poly <vilib>:"DAQmx Write.vi"("task/channels in"=w200, "data"=w180, "error in"=w198) -> ("task out"=w199:refnum<k21>, "error out"=w197:errorcluster)  [unwired: 10 in, 1 out]
        n112 = call <vilib>:"DAQmx Clear Task.vi"("task in"=w199, "error in"=w197) -> ("error out"=→"error out 42":errorcluster)  [unwired: 13 in]
        n113 = call-poly <vilib>:"DAQmx Create Virtual Channel.vi"("lines"=tag "myDAQ1/port0/line2") -> ("task out"=w194:refnum<k21>, "error out"=w192:errorcluster)  [unwired: 13 in]
        n114 = call "Stall Data Flow.vim"("value in"=bool[] [TRUE], "milliseconds to wait"=333) -> ("value out"=w178:bool[])  [unwired: 1 out]
        n115 = call-poly <vilib>:"DAQmx Write.vi"("task/channels in"=w194, "data"=w178, "error in"=w192) -> ("task out"=w193:refnum<k21>, "error out"=w191:errorcluster)  [unwired: 10 in, 1 out]
        n116 = call <vilib>:"DAQmx Clear Task.vi"("task in"=w193, "error in"=w191) -> ("error out"=→"error out 43":errorcluster)  [unwired: 13 in]
        n117 = call-poly <vilib>:"DAQmx Create Virtual Channel.vi"("lines"=tag "myDAQ1/port0/line4") -> ("task out"=w188:refnum<k21>, "error out"=w186:errorcluster)  [unwired: 13 in]
        n118 = call "Stall Data Flow.vim"("value in"=bool[] [TRUE], "milliseconds to wait"=655) -> ("value out"=w175:bool[])  [unwired: 1 out]
        n119 = call-poly <vilib>:"DAQmx Write.vi"("task/channels in"=w188, "data"=w175, "error in"=w186) -> ("task out"=w187:refnum<k21>, "error out"=w185:errorcluster)  [unwired: 10 in, 1 out]
        n120 = call <vilib>:"DAQmx Clear Task.vi"("task in"=w187, "error in"=w185) -> ("error out"=→"error out 44":errorcluster)  [unwired: 13 in]
      }
      frame "v4 S" {
        n121 = call-poly <vilib>:"DAQmx Create Virtual Channel.vi"("lines"=tag "myDAQ1/port0/line0:7") -> ("task out"=w207:refnum<k21>, "error out"=w205:errorcluster)  [unwired: 13 in]
        n122 = call-poly <vilib>:"DAQmx Write.vi"("task/channels in"=w207, "data"=bool[] [FALSE, FALSE, FALSE, FALSE, TRUE, TRUE, TRUE, TRUE], "error in"=w205) -> ("task out"=w206:refnum<k21>, "error out"=w204:errorcluster)  [unwired: 10 in, 1 out]
        n123 = call <vilib>:"DAQmx Clear Task.vi"("task in"=w206, "error in"=w204) -> ("error out"=→"error out 50":errorcluster)  [unwired: 13 in]
      }
      frame "v4 L" {
        n124 = call-poly <vilib>:"DAQmx Create Virtual Channel.vi"("lines"=tag "myDAQ1/port0/line0:7") -> ("task out"=w214:refnum<k21>, "error out"=w212:errorcluster)  [unwired: 13 in]
        n125 = call-poly <vilib>:"DAQmx Write.vi"("task/channels in"=w214, "data"=bool[] [TRUE, TRUE, TRUE, TRUE, FALSE, FALSE, FALSE, FALSE], "error in"=w212) -> ("task out"=w213:refnum<k21>, "error out"=w211:errorcluster)  [unwired: 10 in, 1 out]
        n126 = call <vilib>:"DAQmx Clear Task.vi"("task in"=w213, "error in"=w211) -> ("error out"=→"error out 49":errorcluster)  [unwired: 13 in]
      }
      frame "v4 double" {
        n127 = call-poly <vilib>:"DAQmx Create Virtual Channel.vi"("lines"=tag "myDAQ1/port0/line0:7") -> ("task out"=w221:refnum<k21>, "error out"=w219:errorcluster)  [unwired: 13 in]
        n128 = call-poly <vilib>:"DAQmx Write.vi"("task/channels in"=w221, "data"=bool[] [FALSE, FALSE, FALSE, FALSE, FALSE, FALSE, FALSE, FALSE], "error in"=w219) -> ("task out"=w220:refnum<k21>, "error out"=w218:errorcluster)  [unwired: 10 in, 1 out]
        n129 = call <vilib>:"DAQmx Clear Task.vi"("task in"=w220, "error in"=w218) -> ("error out"=→"error out 48":errorcluster)  [unwired: 13 in]
      }
      frame "v4 E" {
        n130 = call-poly <vilib>:"DAQmx Create Virtual Channel.vi"("lines"=tag "myDAQ1/port0/line0:7") -> ("task out"=w228:refnum<k21>, "error out"=w226:errorcluster)  [unwired: 13 in]
        n131 = call-poly <vilib>:"DAQmx Write.vi"("task/channels in"=w228, "data"=bool[] [TRUE, TRUE, FALSE, FALSE, FALSE, FALSE, TRUE, TRUE], "error in"=w226) -> ("task out"=w227:refnum<k21>, "error out"=w225:errorcluster)  [unwired: 10 in, 1 out]
        n132 = call <vilib>:"DAQmx Clear Task.vi"("task in"=w227, "error in"=w225) -> ("error out"=→"error out 47":errorcluster)  [unwired: 13 in]
      }
      frame "v4 B" {
        n133 = call-poly <vilib>:"DAQmx Create Virtual Channel.vi"("lines"=tag "myDAQ1/port0/line0:7") -> ("task out"=w235:refnum<k21>, "error out"=w233:errorcluster)  [unwired: 13 in]
        n134 = call-poly <vilib>:"DAQmx Write.vi"("task/channels in"=w235, "data"=bool[] [TRUE, TRUE, FALSE, FALSE, FALSE, FALSE, FALSE, FALSE], "error in"=w233) -> ("task out"=w234:refnum<k21>, "error out"=w232:errorcluster)  [unwired: 10 in, 1 out]
        n135 = call <vilib>:"DAQmx Clear Task.vi"("task in"=w234, "error in"=w232) -> ("error out"=→"error out 46":errorcluster)  [unwired: 13 in]
      }
    }
  }
  n136 = Current VI's Path() -> (path=w8:path)
  n137 = Build Path(base path=w8, name or relative path=path "../Jingle Bells.wav" ("Sound File Path")) -> (appended path=w9:path)
  n138 = call-poly <vilib>:"Sound File Info.vi"("path"=w9) -> ("error out"=w22:errorcluster, "sound format"=w14:T4, "path out"=w15:path)  [unwired: 7 in, 1 out]
  n139 = call-poly <vilib>:"Sound File Open.vi"("error in (no error)"=w22, "path"=w15) -> ("error out"=w21:errorcluster, "sound file refnum"=w23:T5)  [unwired: 8 in]
  n140 = call <vilib>:"Sound Output Configure.vi"("number of samples/ch"="Number of Samples/Iteration", "sample mode"=w12, "error in (no error)"=w21, "sound format"=w14, "device ID"="Device ID") -> ("error out"=w20:errorcluster, "task ID"=w27:T6)  [unwired: 5 in]
  n141 = while {
    tunnel: "Number of Samples/Iteration" -> [w384]
    tunnel: w23 -> [w391]
    tunnel: [w390] -> w25
    tunnel: w20 -> [w392]
    tunnel: [w383] -> w24
    tunnel: w27 -> [w389]
    tunnel: [w393] -> w18
    i -> [w366]
    stop <- w385 stop-if-true
    # "Read the specified number of samples from the file. Write data read from the file to the sound output device."
    # "Read Sound File and Generate Sound"
    n142 = Greater?(x=w366, y=530) -> (0:w364:bool)
    n143 = call-poly <vilib>:"Sound File Read.vi"("number of samples/ch (-1: all)"=w384, "error in (no error)"=w392, "sound file refnum"=w391) -> ("error out"=w388:errorcluster, "data"=w381:waveform(dbl)[], "sound file refnum out"=w390:T5, "end of file?"=w386:bool)  [unwired: 4 in, 1 out]
    "Array 3" <- w381
    "Waveform Chart" <- w381
    n144 = call-poly <vilib>:"Sound Output Write.vi"("error in (no error)"=w388, "data"=w381, "task ID"=w389) -> ("error out"=w383:errorcluster, "task ID out"=w393:T6)  [unwired: 7 in]
    n145 = Compound Arithmetic op=OR(w383, w386, "Stop") -> (w385:bool)
    n146 = call-poly <vilib>:"DAQmx Create Virtual Channel.vi"("lines"=tag "myDAQ1/port0/line0:7") -> ("task out"=w375:refnum<k21>, "error out"=w373:errorcluster)  [unwired: 13 in]
    n147 = call <vilib>:"Waveform Min Max.vi"() -> ()  [unwired: 6 in, 6 out]
    n148 = Index Array(array=w381, index=1) -> (element=w377:waveform(dbl))
    n149 = Greater?(x=w377, y=0.1) -> (0:w379:bool[])
    n150 = Greater?(x=-0.1, y=w377) -> (0:w376:bool[])
    n151 = Or(x=w376, y=w379) -> (x .or. y?=w368:bool[])
    "Array 7" <- w368
    n152 = Reshape Array(w368, 8) -> (w367:bool[])
    n153 = call-poly <vilib>:"DAQmx Write.vi"("task/channels in"=w375, "auto start"=w364, "data"=w367, "error in"=w373) -> ("task out"=w374:refnum<k21>, "error out"=w372:errorcluster)  [unwired: 9 in, 1 out]
    n154 = call <vilib>:"DAQmx Clear Task.vi"("task in"=w374, "error in"=w372) -> ("error out"=→"error out 38":errorcluster)  [unwired: 13 in]
    "Current Iteration" <- w366
  }
  n155 = call <vilib>:"Sound File Close.vi"("error in (no error)"=w24, "sound file refnum"=w25) -> ("error out"=w17:errorcluster)  [unwired: 9 in]
  n156 = call <vilib>:"Sound Output Wait.vi"("error in (no error)"=w17, "task ID"=w18) -> ("error out"=w16:errorcluster, "task ID out"=w19:T6)  [unwired: 8 in]
  n157 = call <vilib>:"Sound Output Clear.vi"("error in (no error)"=w16, "task ID"=w19) -> ("error out"=w11:errorcluster)  [unwired: 9 in]
  n158 = call <vilib>:"Simple Error Handler.vi"("error in (no error)"=w11) -> ()  [unwired: 4 in, 5 out]
